vi "Initialize MeasurementLink Session.vi"(7 "remote connection options":T2, 8 "error in":errorcluster, 9 "initialize and close session behavior":T1, 10 "session initialization details":T3, 11 "instrument in":refnum<class "Instrument.lvclass">) -> (0 "error out":errorcluster, 2 "session out":variant, 3 "instrument out":refnum<class "Instrument.lvclass">)   [LabVIEW 2020, in "MeasurementLink niScope.lvlib" / "Instrument.lvclass"]
uses:
  Instrument.lvclass
  MeasurementLink Instrument/IInstrument/Remote Connection Options.ctl
  MeasurementLink Instrument/IInstrument/Initialize and Close Session Behavior.ctl
  Instrument.lvclass/Instrument.ctl
  MeasurementLink Measurement Server/Helpers/Error Strings Global Internal.vi
  MeasurementLink Instrument/IInstrument/IInstrument.lvclass
  MeasurementLink Instrument/IInstrument/Session Initialization Details.ctl
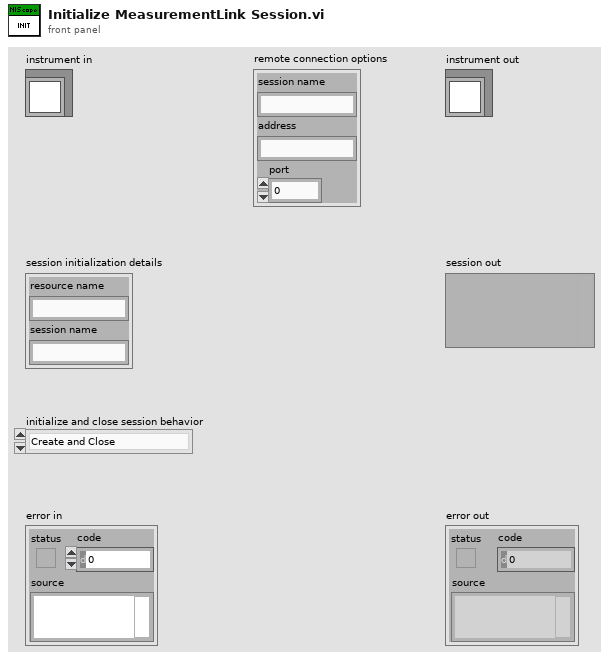
[diagram p1: front panel]
types:
  T1 = typedef "MeasurementLink Instrument.lvlib/IInstrument.lvclass/Initialize and Close Session Behavior.ctl" = enum16{"Create and Close", "Attach and Detach", "Create and Detach", "Attach and Close"}
  T2 = typedef "MeasurementLink Instrument.lvlib/IInstrument.lvclass/Remote Connection Options.ctl" = cluster{"session name":string, "address":string, "port":u32}
  T3 = typedef "MeasurementLink Instrument.lvlib/IInstrument.lvclass/Session Initialization Details.ctl" = cluster{"resource name":string, "session name":string}
  T4 = typedef "MeasurementLink Instrument.lvlib/IInstrument.lvclass/Initialize Session Behavior.ctl" = enum16{"Create Session", "Attach Session"}
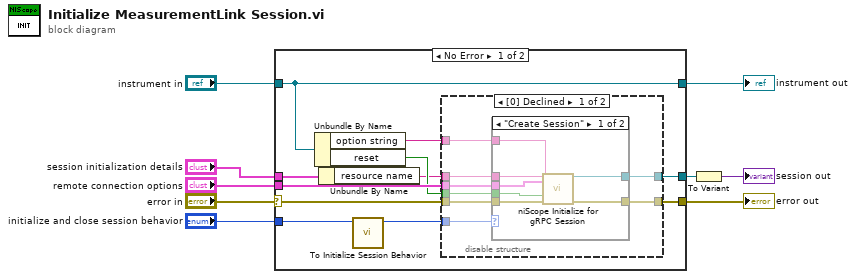
[diagram p0: block diagram]
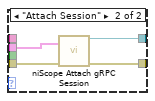
[diagram p2: hidden frame]
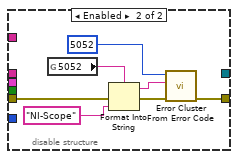
[diagram p3: hidden frame]
diagram:
  n1 = case shown="No Error" "error in" {
    selector: "error in" -> [w17 w47]
    tunnel: [w16 w47] -> w8
    tunnel: "instrument in" -> [w14 w48]
    tunnel: [w14 w48] -> w6
    tunnel: "initialize and close session behavior" -> [w20 _]
    tunnel: "remote connection options" -> [w19 _]
    tunnel: "session initialization details" -> [w15 _]
    tunnel: [w18 _] -> w2
    frame No Error {
      n2 = Unbundle By Name(w14) -> ("option string"=w13:string, "reset"=w12:bool)
      n3 = Unbundle By Name(w15) -> ("resource name"=w10:string)
      n4 = call "To Initialize Session Behavior.vi"("initialize and close session behavior"=w20) -> ("initialize session behavior"=w11:T4)  [unwired: 10 in]
      n5 = disable-structure shown="[0] Declined" {
        disable-tunnel: w11 -> [w28 _]
        disable-tunnel: w19 -> [w27 _]
        disable-tunnel: [w26 _] -> w18
        disable-tunnel: w17 -> [w25 w41]
        disable-tunnel: [w24 w40] -> w16
        disable-tunnel: w10 -> [w23 _]
        disable-tunnel: w13 -> [w22 _]
        disable-tunnel: w12 -> [w21 _]
        frame Disabled {
          n6 = case shown="\"Create Session\"" w28 {
            tunnel: w27 -> [w34 w39]
            tunnel: [w33 w38] -> w26
            tunnel: w25 -> [w35 w37]
            tunnel: [w32 w36] -> w24
            tunnel: w23 -> [w31 _]
            tunnel: w22 -> [w30 _]
            tunnel: w21 -> [w29 _]
            frame "Create Session" {
              n7 = call <instrlib>:"niScope Initialize for gRPC Session.vi"("resource name"=w31, "gRPC options"=w34, "option string"=w30, "reset device"=w29, "error in"=w35) -> ("instrument handle"=w33:refnum<k15>, "error out"=w32:errorcluster)  [unwired: 9 in]
            }
            frame "Attach Session" {
              n8 = call <instrlib>:"niScope Attach gRPC Session.vi"("gRPC options"=w39, "error in"=w37) -> ("instrument handle"=w38:refnum<k15>, "error out"=w36:errorcluster)  [unwired: 12 in]
            }
          }
        }
        frame Enabled {
          n9 = global read "Error Strings Global Internal.vi" "5052"() -> (w45:string)
          n10 = Format Into String(format string=w45, error in=w41, "NI-Scope") -> (resulting string=w42:string, error out=w43:errorcluster)  [unwired: 1 in]
          n11 = call <vilib>:"Error Cluster From Error Code.vi"("error in (no error)"=w43, "error message (\"\")"=w42, "error code (0)"=5052) -> ("error out"=w40:errorcluster)  [unwired: 6 in]
        }
      }
    }
    frame Error {
    }
  }
  "error out" <- w8
  "instrument out" <- w6
  n12 = To Variant(anything=w2) -> (Variant=→"session out":variant)
